vi "time_delta.vi"() -> (0 "dt (s)":dbl)   [LabVIEW 2016, in "ArgosLib.lvlib"]
uses:
  ArgosLib.lvlib
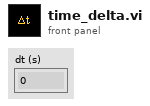
[diagram p1: front panel]
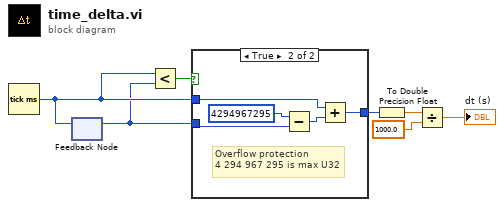
[diagram p0: block diagram]
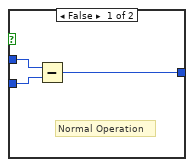
[diagram p2: hidden frame]
diagram:
  n1 = Tick Count (ms)() -> (millisecond timer value=w6:u32)
  n2 = feedback-in #1(w6) -> ()
  n3 = feedback #1() -> (w5:u32)  [unwired: 1 in]
  n4 = Less?(x=w6, y=w5) -> (x < y?=w7:bool)
  n5 = case shown="True" w7 {
    tunnel: w6 -> [w10 w12]
    tunnel: w5 -> [w9 w14]
    tunnel: [w8 w11] -> w2
    frame False {
      # "Normal Operation"
      n6 = Subtract(x=w10, y=w9) -> (x-y=w8:u32)
    }
    frame True {
      # "Overflow protection\n4 294 967 295 is max U32"
      n7 = Subtract(x=u32 4294967295, y=w14) -> (x-y=w13:u32)
      n8 = Add(x=w12, y=w13) -> (x+y=w11:u32)
    }
  }
  n9 = To Double Precision Float(number=w2) -> (double precision float=w1:dbl)
  n10 = Divide(x=w1, y=1000.0) -> (x/y=→"dt (s)":dbl)
